vi "libresult_ready.vi"(8 "error in (no error)":errorcluster, 10 "id":string, 11 "input":i32) -> (0 "error out":errorcluster, 2 "is":bool)   [LabVIEW 2015]
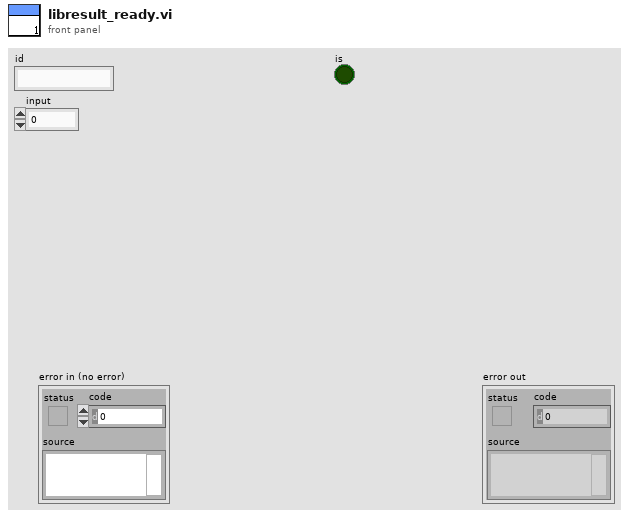
[diagram p1: front panel]
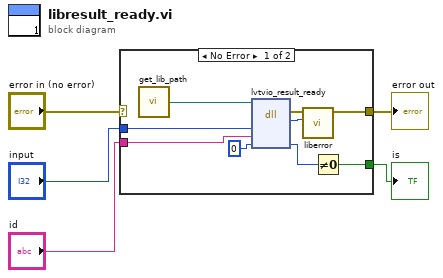
[diagram p0: block diagram]
diagram:
  n1 = case shown="No Error" "error in (no error)" {
    selector: "error in (no error)" -> [_ w15]
    tunnel: [w6 w15] -> w4
    tunnel: [w11 _] -> w3
    tunnel: "id" -> [w10 _]
    tunnel: "input" -> [w9 _]
    frame No Error {
      n2 = call "get_lib_path.vi"() -> ("Path"=w14:path)
      n3 = dll-call lib="S:/thingiverselv/lib/liblvtvio.dll" fn="lvtvio_result_ready"(path in=w14, "input"=w9, "id"=w10, "is"=0) -> (error out=w7:errorcluster, "return type"=w8:i32, "is"=w12:i32)  [unwired: 4 in, 1 out]
      n4 = call "liberror.vi"("tvio errors"=w8, "error in (no error)"=w7) -> ("error out"=w6:errorcluster)  [unwired: 9 in]
      n5 = Not Equal To 0?(x=w12) -> (x != 0?=w11:bool)
    }
    frame Error {
    }
  }
  "error out" <- w4
  "is" <- w3
